vi "Write VI Path.vi"(8 "error in (no error)":errorcluster, 10 "VI Path":path, 11 "VI in":refnum<class "VI.lvclass">) -> (0 "error out":errorcluster, 3 "VI out":refnum<class "VI.lvclass">)   [LabVIEW 2019, in "VI.lvclass"]
uses:
  VI.lvclass
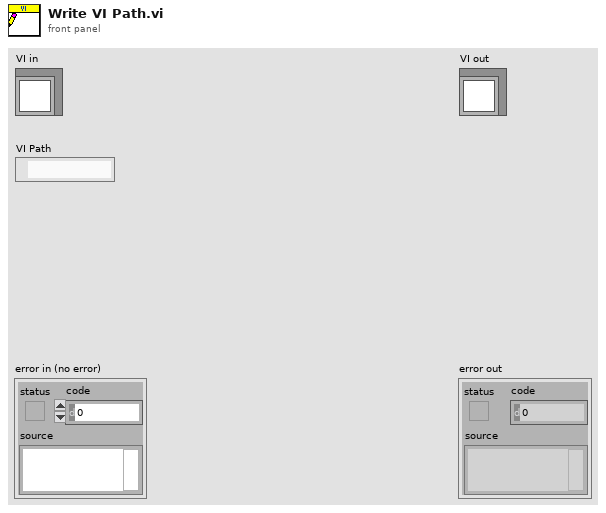
[diagram p1: front panel]
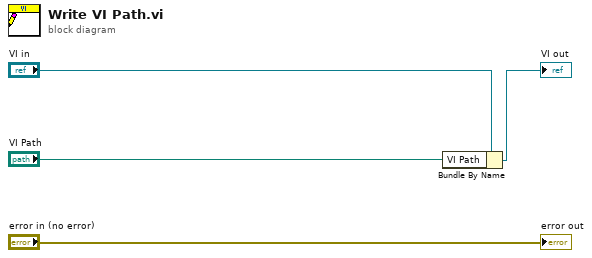
[diagram p0: block diagram]
diagram:
  n1 = Bundle By Name(cluster="VI in", "VI Path"="VI Path") -> (→"VI out":refnum<class "VI.lvclass">)
  "error out" <- "error in (no error)"
